vi "IMULoop.vi"(6 "I2CDevRef 2":T10={"DevStatus"={"status"=FALSE, "code"=0, "source"=""}, "Controller"=enum."Controller 1", "Device Address"=0, "Handle"=0, "I2C Bus"=enum."Invalid"} {"Device Address" format="%.0x"}, 8 "AccelerometerDevRef":T1={"DevStatus"={"status"=FALSE, "code"=0, "source"=""}, "Controller"=enum."Controller 1", "Scaling"={"Gain (VoltsPerG)"=0.0, "Center Voltage"=0.0}, "Analog Channels"={"X-Axis"=enum."Invalid", "Y-Axis"=enum."Invalid", "Z-Axis"=enum."Invalid"}, "I2C Bus"=enum."Invalid", "SPI Bus"=enum."Invalid", "Accel Range"=0, "ADXL345 Axes"={"X-Axis"=FALSE, "Y-Axis"=FALSE, "Z-Axis"=FALSE}, "Handle"=0, "Device Address"=0, "Accel Type"=enum."Analog"} {"Device Address" format="%.0x"; "Accel Range" items=["+/- 2 g", "+/- 4 g", "+/- 8 g", "+/- 16 g"]}) -> ()   [LabVIEW 2014]
uses:
  <vilib>/Rock Robotics/WPI/I2C/WPI_I2CDevRef.ctl
  <vilib>/Rock Robotics/SystemInterfaces/Typedef/FPGA_TypedefDigitalModule.ctl
  <vilib>/Rock Robotics/SystemInterfaces/i2clib/i2c_bus.ctl
  <vilib>/Rock Robotics/WPI/Accelerometer/WPI_AccelerometerDevRef.ctl
  <vilib>/Rock Robotics/SystemInterfaces/Typedef/FPGA_TypedefAnalogModule.ctl
  <vilib>/Rock Robotics/WPI/Accelerometer/WPI_AccelerometerScaling.ctl
  <vilib>/Rock Robotics/WPI/Accelerometer/WPI_AccelerometerAnalogChannels.ctl
  <vilib>/Rock Robotics/SystemInterfaces/AI/FPGA_AIChannel.ctl
  <vilib>/Rock Robotics/SystemInterfaces/spilib/spi_bus.ctl
  <vilib>/Rock Robotics/WPI/Accelerometer/ADXL345 Range.ctl
  <vilib>/Rock Robotics/WPI/Accelerometer/WPI_AccelerometerADXL345 Axes.ctl
  <vilib>/Platform/TimedLoop/XDataNode/timing_clust.ctl
  <vilib>/Platform/TimedLoop/XDataNode/nitl_modes.ctl
  <vilib>/Platform/TimedLoop/XDataNode/wakeup.ctl
  Common Code/IMU Data.ctl
  Robot Global Data.vi
  <vilib>/Platform/TimedLoop/XDataNode/XDataNode.xnode
  <vilib>/Platform/TimedLoop/XDataNode/XDNodeRunTimeDep.lvlib
panel:
  # "ADXL345"
  # "Analog"
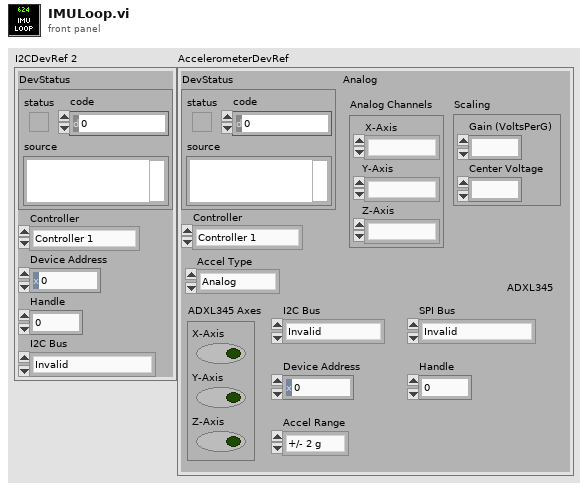
[diagram p1: front panel]
types:
  T1 = typedef "WPI_AccelerometerDevRef.ctl" = cluster{"DevStatus":errorcluster, "Controller":T2, "Scaling":T3, "Analog Channels":T4, "I2C Bus":T6, "SPI Bus":T7, "Accel Range":T8, "ADXL345 Axes":T9, "Handle":i32, "Device Address":u8, "Accel Type":enum16{"Analog", "ADXL345 I2C", "ADXL345 SPI", "Internal"}}
  T2 = typedef "FPGA_TypedefAnalogModule.ctl" = enum16{"Controller 1"}
  T3 = typedef "WPI_AccelerometerScaling.ctl" = cluster{"Gain (VoltsPerG)":dbl, "Center Voltage":dbl}
  T4 = typedef "WPI_AccelerometerAnalogChannels.ctl" = cluster{"X-Axis":T5, "Y-Axis":T5, "Z-Axis":T5}
  T5 = typedef "FPGA_AIChannel.ctl" = enum8{"AI 0", "AI 1", "AI 2", "AI 3", "AI MXP 0", "AI MXP 1", "AI MXP 2", "AI MXP 3", "Invalid"}
  T6 = typedef "i2c_bus.ctl" = enum16{"I2C On-Board", "I2C MXP", "Invalid"}
  T7 = typedef "spi_bus.ctl" = enum16{"SPI On-Board, CS0", "SPI On-Board, CS1", "SPI On-Board, CS2", "SPI On-Board, CS3", "SPI MXP", "Invalid"}
  T8 = typedef "ADXL345 Range.ctl" = u8
  T9 = typedef "WPI_AccelerometerADXL345 Axes.ctl" = cluster{"X-Axis":bool, "Y-Axis":bool, "Z-Axis":bool}
  T10 = typedef "WPI_I2CDevRef.ctl" = cluster{"DevStatus":errorcluster, "Controller":T11, "Device Address":u8, "Handle":i32, "I2C Bus":T6}
  T11 = typedef "FPGA_TypedefDigitalModule.ctl" = enum16{"Controller 1"}
  T12 = typedef "IMU Data.ctl" = cluster{"Pitch":sgl, "Roll":sgl, "Yaw":sgl}
  T13 = typedef "XDNodeRunTimeDep.lvlib/timing_clust.ctl" = cluster{"Expected End [f-1]":u64, "Actual End [f-1]":u64, "Finished Late? [f-1]":bool, "Expected End [i-1]":u64, "Actual End [i-1]":u64, "Finished Late? [i-1]":bool, "Expected Start [i]":u64, "Actual Start [i]":u64, "Expected Start [f]":u64, "Actual Start [f]":u64, "Source Name":string, "Structure Name":string, "Period":i64, "Deadline":i64, "Offset":i64, "Start":i64, "Priority":i32, "Timeout":i32, "Mode":T14, "Wakeup Reason":T15, "Error":errorcluster, "Source Type":string, "Secondary Source Type":string, "Global End Time":u64, "Global Start Time":u64, "Frame Duration":u64, "Iteration Duration":u64, "Assigned CPU":i32, "I/O Scan Engine Mode":u32}
  T14 = typedef "XDNodeRunTimeDep.lvlib/nitl_modes.ctl" = enum32{"No Change", "Process missed periods, maintain original phase", "Discard missed periods, maintain original phase", "Process missed periods, ignore original phase", "Discard missed periods, ignore original phase"}
  T15 = typedef "XDNodeRunTimeDep.lvlib/wakeup.ctl" = enum32{"Normal", "Aborted", "Asynchronous wakeup", "Timing source error", "Timed loop error", "Timeout"}
  T16 = cluster{"X-Axis":dbl, "Y-Axis":dbl, "Z-Axis":dbl}
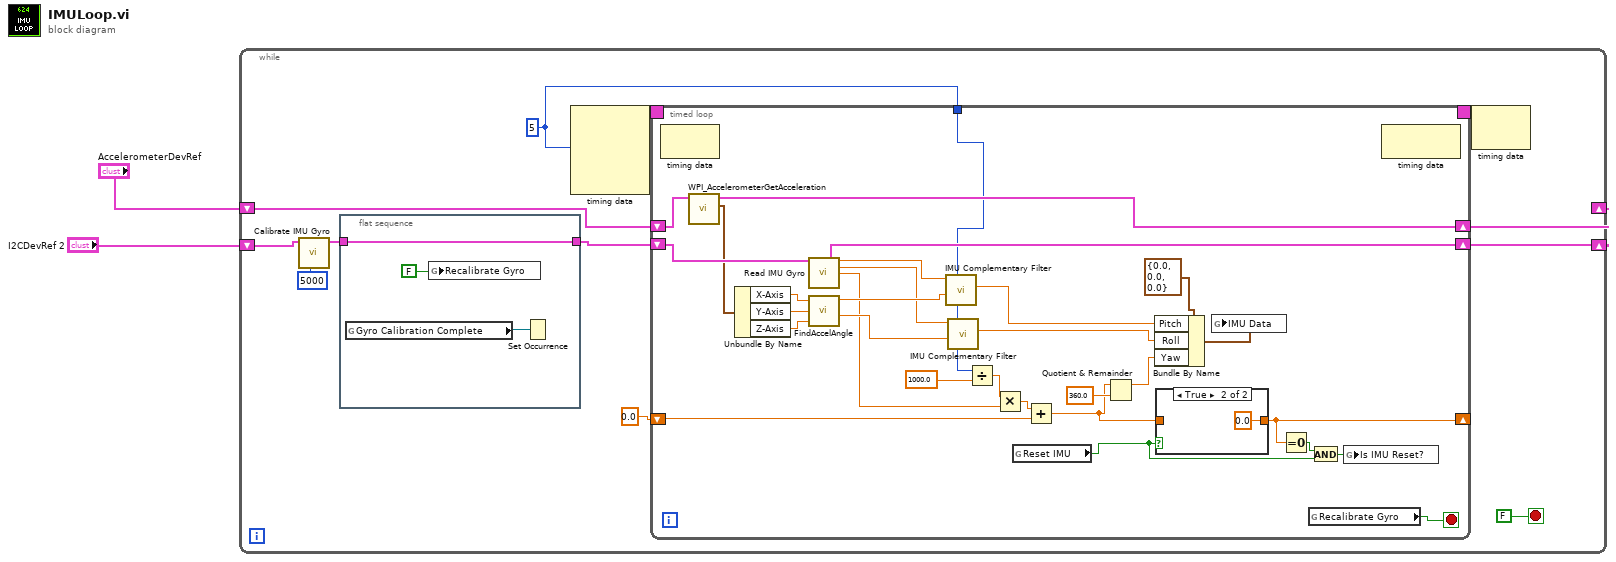
[diagram p0: block diagram]
diagram:
  n1 = while {
    shift-right: [w7] -> _
    shift-left: "I2CDevRef 2" -> [w8]
    shift-right: [w6] -> _
    shift-left: "AccelerometerDevRef" -> [w12]
    stop <- FALSE stop-if-true
    w11 = u16 5 ("Period")
    n2 = call "Calibrate IMU Gyro.vi"("Calib time (ms)"=u32 5000, "I2CDevRef in"=w8) -> ("I2CDevRef out"=w4:T10)  [unwired: 9 in]
    n3 = flat-sequence {
      tunnel: [w17] -> w3
      tunnel: w4 -> [w17]
      frame #0 {
        n4 = global read "Robot Global Data.vi" "Gyro Calibration Complete"() -> (w15:refnum<k4>)
        n5 = global write "Robot Global Data.vi" "Recalibrate Gyro"(FALSE ("Recalibrate Gyro")) -> ()
        n6 = Set Occurrence(w15) -> ()
      }
    }
    n7 = node-c288(w11) -> (w14:T13)  [unwired: 3 in]
    n8 = timed-loop {
      timing: w14 -> [_]
      timing-out: [_] -> w13
      shift-right: [w47] -> w7
      shift-left: w3 -> [w46]
      shift-right: [w44] -> w6
      shift-left: w12 -> [w45]
      tunnel: w11 -> [w42]
      shift-right: [w22] -> _
      shift-left: 0.0 -> [w43]
      stop <- w18 stop-if-true
      n9 = node-c288() -> ()  [unwired: 1 in, 1 out]
      n10 = call <vilib>:"WPI_AccelerometerGetAcceleration.vi"("AccelerometerDevRef"=w45) -> ("Accelerations"=w38:T16, "AccelerometerDevRef"=w44:T1)  [unwired: 8 in, 1 out]
      n11 = Unbundle By Name(w38) -> ("X-Axis"=w39:dbl, "Y-Axis"=w40:dbl, "Z-Axis"=w41:dbl)
      n12 = call "Read IMU Gyro.vi"("I2CDevRef"=w46) -> ("I2CDevRef 2"=w47:T10, "X"=w37:dbl, "Y"=w35:dbl, "Z"=w31:dbl)  [unwired: 8 in, 3 out]
      n13 = call "FindAccelAngle.vi"("Z"=w41, "Y"=w40, "X"=w39) -> ("Roll"=w34:dbl, "Pitch"=w36:dbl)  [unwired: 4 in]
      n14 = call "IMU Complementary Filter.vi"("dt (ms)"=w42, "Accelerometer Angle"=w36, "Angular vel (gyro, deg/sec)"=w37) -> ("Current Angle"=w26:dbl)  [unwired: 8 in]
      n15 = call "IMU Complementary Filter.vi"("dt (ms)"=w42, "Accelerometer Angle"=w34, "Angular vel (gyro, deg/sec)"=w35) -> ("Current Angle"=w27:dbl)  [unwired: 8 in]
      n16 = Divide(x=w42, y=1000.0) -> (x/y=w32:dbl)
      n17 = Multiply(x=w32, y=w31) -> (x*y=w30:dbl)
      n18 = global read "Robot Global Data.vi" "Reset IMU"() -> (w19:bool)
      n19 = Add(x=w30, y=w43) -> (x+y=w23:dbl)
      n20 = Quotient & Remainder(x=w23, y=360.0) -> (x-y*floor(x/y)=w24:dbl)  [unwired: 1 out]
      n21 = Bundle By Name(cluster=T12 {"Pitch"=0.0, "Roll"=0.0, "Yaw"=0.0} ("IMU Data"), "Pitch"=w26, "Roll"=w27, "Yaw"=w24) -> (w28:T12)
      n22 = case shown="True" w19 {
        tunnel: w23 -> [w48 _]
        tunnel: [w48 0.0] -> w22
        frame False {
        }
        frame True {
        }
      }
      n23 = global write "Robot Global Data.vi" "IMU Data"(w28) -> ()
      n24 = Equal To 0?(x=w22) -> (x = 0?=w20:bool)
      n25 = global read "Robot Global Data.vi" "Recalibrate Gyro"() -> (w18:bool)
      n26 = And(x=w20, y=w19) -> (x .and. y?=w21:bool)
      n27 = global write "Robot Global Data.vi" "Is IMU Reset?"(w21) -> ()
      n28 = node-c288() -> ()  [unwired: 1 in, 1 out]
    }
    n29 = node-c288(w13) -> ()  [unwired: 1 out]
  }
